vi "Square_axis.vi"(1 "axis":dbl) -> (0 "axis squared":dbl)   [LabVIEW 2013]
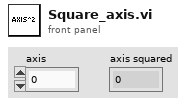
[diagram p1: front panel]
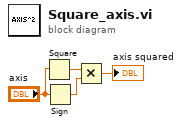
[diagram p0: block diagram]
diagram:
  n1 = Square(x="axis") -> (x^2=w1:dbl)
  n2 = Sign(1:"axis") -> (0:w2:dbl)
  n3 = Multiply(x=w1, y=w2) -> (x*y=→"axis squared":dbl)
